vi "SPD.QE&DCR Meas.vi"(8 "Error In":errorcluster, 11 "SPD.Stand Ctrl in":T1 {"spdDeviceSession"."hidSPD.Controller"."HV_bias" format="%#_6p, V"; "spdDeviceSession"."hidSPD.Controller"."TSet" format="%#_6p, DegC"}) -> (0 "Error Out":errorcluster, 1 "QE":dbl, 2 "DCR":dbl, 3 "SPD.Stand Ctrl out":T1 {"spdDeviceSession"."hidSPD.Controller"."HV_bias" format="%#_6p, V"; "spdDeviceSession"."hidSPD.Controller"."TSet" format="%#_6p, DegC"})   [LabVIEW 2018]
uses:
  typedefs/SPD.Stand Ctrl.ctl
  Instruments/SPD HID Interface/hidSPDLibForLabView/LibVIs/hidSPD Controls/hidSPD Device Session.ctl
  Instruments/SPD HID Interface/hidSPDLibForLabView/LibVIs/hidSPD Controls/hidSPD Controller.ctl
  Instruments/KC705 DevBoard/typedefs/DevB.Session.ctl
  Instruments/KeySight 53230A/typedefs/FreqC.Session.ctl
  Instruments/KeySight 8164B/KeySight 8164B LAN InstrLib/typedefs/KeySight 8164B control.ctl
  Instruments/LeCroy SDA830/typedefs/LeCroy.Session.ctl
  typedefs/SPD.Events.ctl
  <vilib>/Utility/config.llb/Config Data RefNum.ctl
  typedefs/SPD.Meas Result.ctl
  02_Strobe_Phase Test/SPD.Strobe_Phase Test Limits.ctl
  Instruments/KeySight 8164B/KeySight 8164B LAN InstrLib.lvlib
  Instruments/SPD HID Interface/hidSPDLibForLabView/hidSPDLibForLabView.lvlib
  <vilib>/Utility/config.llb/NI_LVConfig.lvlib
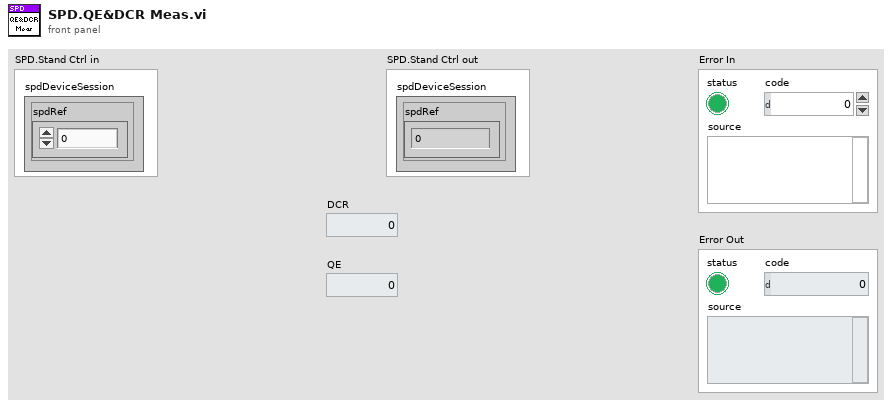
[diagram p1: front panel]
types:
  T1 = typedef "SPD.Stand Ctrl.ctl" = cluster{"spdDeviceSession":T2, "DevBSession":T4, "FreqCSession":T5, "8164BSession":T6, "LeCroySession":T7, "Events":T8, "configFile":T9, "SPD.Result":T10}
  T2 = typedef "hidSPDLibForLabView.lvlib/hidSPD Device Session.ctl" = cluster{"spdRef":u64, "connected":bool, "spdName":string, "hidSPD.Controller":T3}
  T3 = typedef "hidSPDLibForLabView.lvlib/hidSPD Controller.ctl" = cluster{"TSet":sgl, "HV_bias":sgl, "DDS_stb_code":u16}
  T4 = typedef "DevB.Session.ctl" = cluster{"DevBRef":refnum<visa-resource-name>, "connected":bool}
  T5 = typedef "FreqC.Session.ctl" = cluster{"FreqCRef":refnum<visa-resource-name>, "timeout":dbl, "Gate":dbl, "connected":bool}
  T6 = typedef "KeySight 8164B LAN InstrLib.lvlib/KeySight 8164B control.ctl" = cluster{"Connection ID":refnum<k5>, "Connected":bool, "Info":string, "Slots Info":string[]}
  T7 = typedef "LeCroy.Session.ctl" = cluster{"LeCroySession":refnum<visa-resource-name>, "connected":bool}
  T8 = typedef "SPD.Events.ctl" = cluster{"DCRTest":refnum<user-event>, "Stop":refnum<user-event>}
  T9 = typedef "NI_LVConfig.lvlib/Config Data RefNum.ctl" = refnum<k1>
  T10 = typedef "SPD.Meas Result.ctl" = cluster{"HV_Bias":dbl[][][], "Stb_code":dbl[], "Temprature":dbl[], "Data":dbl[][][][]}
  T11 = typedef "SPD.Strobe_Phase Test Limits.ctl" = cluster{"ph_start":i32, "ph_stop":i32, "ph_step":i32, "gate":dbl, "num of tests":dbl}
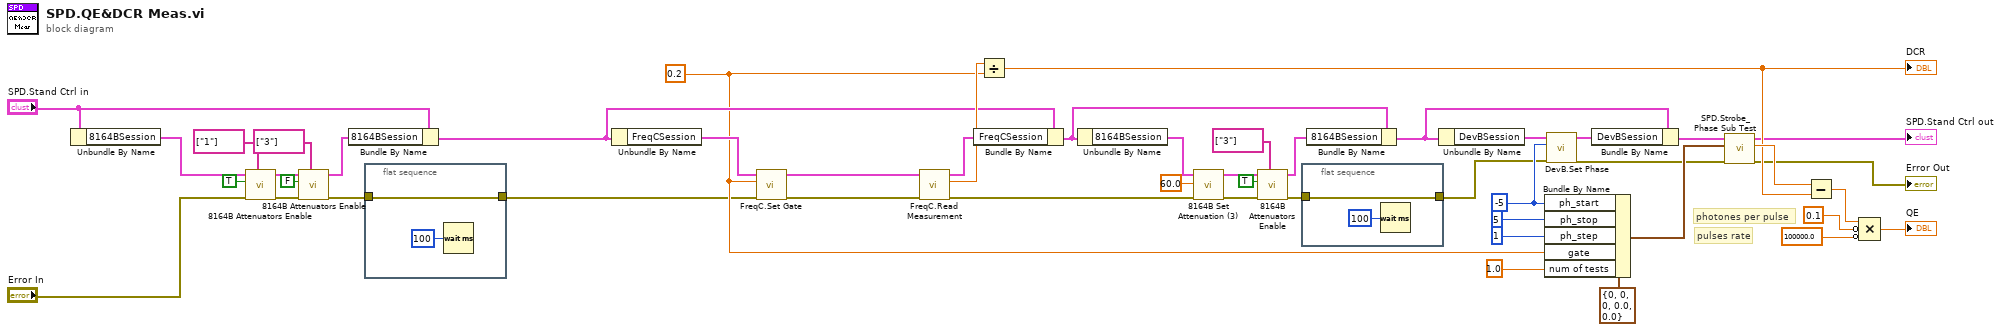
[diagram p0: block diagram]
diagram:
  w30 = -5 ("Phase")
  w27 = 0.2 ("Gate, sec")
  # "pulses rate"
  # "photones per pulse"
  n1 = Unbundle By Name("SPD.Stand Ctrl in") -> ("8164BSession"=w49:T6)
  n2 = call "8164B Attenuators Enable.vi"("Slots"=string[] ["1"], "error in"="Error In", "Enable"=TRUE, "KeySight 8164B control in"=w49) -> ("error out"=w46:errorcluster, "KeySight 8164B control out"=w45:T6)  [unwired: 6 in]
  n3 = call "8164B Attenuators Enable.vi"("Slots"=string[] ["3"], "error in"=w46, "Enable"=FALSE, "KeySight 8164B control in"=w45) -> ("error out"=w4:errorcluster, "KeySight 8164B control out"=w41:T6)  [unwired: 6 in]
  n4 = Bundle By Name(cluster="SPD.Stand Ctrl in", "8164BSession"=w41) -> (w35:T1)
  n5 = flat-sequence {
    tunnel: w4 -> [w51]
    tunnel: [w51] -> w3
    frame #0 {
      n6 = Wait (ms)(milliseconds to wait=u32 100) -> ()  [unwired: 1 out]
    }
  }
  n7 = Unbundle By Name(w35) -> ("FreqCSession"=w39:T5)
  n8 = call "FreqC.Set Gate.vi"("error In"=w3, "Gate, sec"=w27, "FreqC Session in"=w39) -> ("error out"=w37:errorcluster, "FreqC Session out"=w38:T5)  [unwired: 7 in]
  n9 = call "FreqC.Read Measurement.vi"("error In"=w37, "FreqC Session in"=w38) -> ("error out"=w18:errorcluster, "Measurement"=w36:dbl, "FreqC Session out"=w34:T5)  [unwired: 7 in]
  n10 = Bundle By Name(cluster=w35, "FreqCSession"=w34) -> (w13:T1)
  n11 = Divide(x=w36, y=w27) -> (x/y=w21:dbl)
  "DCR" <- w21
  n12 = Unbundle By Name(w13) -> ("8164BSession"=w20:T6)
  n13 = call "8164B Set Attenuation (3).vi"("error in"=w18, "Att 3, dB"=60.0, "KeySight 8164B control in"=w20) -> ("error out"=w14:errorcluster, "KeySight 8164B control out"=w15:T6)  [unwired: 7 in]
  n14 = call "8164B Attenuators Enable.vi"("Slots"=string[] ["3"], "error in"=w14, "Enable"=TRUE, "KeySight 8164B control in"=w15) -> ("error out"=w2:errorcluster, "KeySight 8164B control out"=w12:T6)  [unwired: 6 in]
  n15 = flat-sequence {
    tunnel: w2 -> [w53]
    tunnel: [w53] -> w1
    frame #0 {
      n16 = Wait (ms)(milliseconds to wait=u32 100) -> ()  [unwired: 1 out]
    }
  }
  n17 = Bundle By Name(cluster=w13, "8164BSession"=w12) -> (w11:T1)
  n18 = Unbundle By Name(w11) -> ("DevBSession"=w33:T4)
  n19 = Bundle By Name(cluster=T11 {"ph_start"=0, "ph_stop"=0, "ph_step"=0, "gate"=0.0, "num of tests"=0.0} ("SPD.Strobe_Phase Test Limits"), "ph_start"=w30, "ph_stop"=5, "ph_step"=1, "gate"=w27, "num of tests"=1.0) -> (w24:T11)
  n20 = call "DevB.Set Phase.vi"("error in (no error)"=w1, "Phase"=w30, "DevB Session in"=w33) -> ("error out"=w23:errorcluster, "DevB Session out"=w32:T4)  [unwired: 7 in]
  n21 = Bundle By Name(cluster=w11, "DevBSession"=w32) -> (w25:T1)
  n22 = call "SPD.Strobe_Phase Sub Test.vi"("Error In"=w23, "SPD.Strobe_Phase Test Limits"=w24, "SPD.Stand Ctrl in"=w25) -> ("Error Out"=→"Error Out":errorcluster, "max clicks"=w22:dbl, "SPD.Stand Ctrl out"=→"SPD.Stand Ctrl out":T1)  [unwired: 5 in, 1 out]
  n23 = Subtract(x=w22, y=w21) -> (x-y=w10:dbl)
  n24 = Compound Arithmetic op=MULTIPLY(w10, invert 0.1, invert 100000.0 ("value")) -> (→"QE":dbl)
